vi "upgrade.vi"(7 "tcp conn":refnum<k5>, 10 "application request in":T1, 11 "http responder in":refnum<class "http responder.lvclass">) -> (3 "http responder out":refnum<class "http responder.lvclass">)   [LabVIEW 2016, in "http responder.lvclass"]
uses:
  http responder.lvclass
  HTTP server/http request.ctl
  HTTP server/http method.ctl
  HTTP server/http header data.ctl
  http responder.lvclass/http responder.ctl
  HTTP server/Basic HTTP server.lvclass
  HTTP server/headers/http headers.lvlib
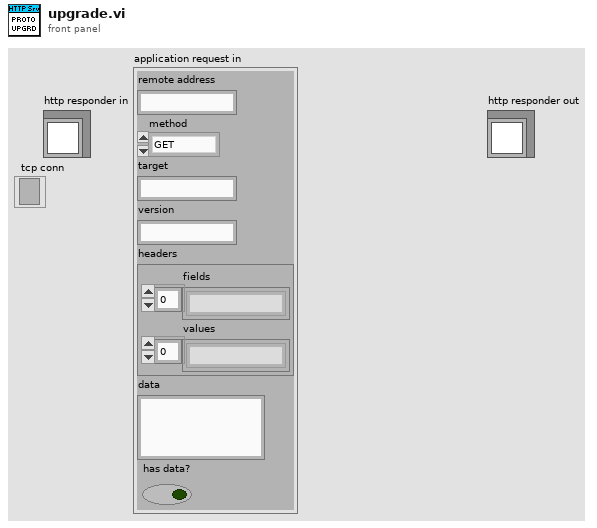
[diagram p1: front panel]
types:
  T1 = typedef "Basic HTTP server.lvclass/http request.ctl" = cluster{"remote address":string, "method":T2, "target":string, "version":string, "headers":T3, "data":string, "has data?":bool}
  T2 = typedef "Basic HTTP server.lvclass/http method.ctl" = enum16{"GET", "POST", "PUT", "DELETE", "HEAD", "OPTIONS", "upgrade"}
  T3 = typedef "http headers.lvlib/http header data.ctl" = cluster{"fields":string[], "values":string[]}
  T4 = typedef "http responder.lvclass/http plugins.ctl" = cluster{"name":string[], "callbacks":T5[]}
  T5 = typedef "http responder.lvclass/http upgrade callback.ctl" = cluster{"callback":refnum<vi>, "parameters":variant, "unregister callback":refnum<vi>}
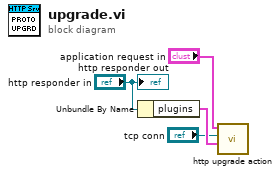
[diagram p0: block diagram]
diagram:
  n1 = Unbundle By Name("http responder in") -> ("plugins"=w3:T4)
  n2 = call "http upgrade action.vi"("plugins"=w3, "tcp conn"="tcp conn", "application request in"="application request in") -> ()  [unwired: 9 in]
  "http responder out" <- "http responder in"
